vi "SimpleLiveAppHistogram.vi"() -> ()   [LabVIEW 2018]
uses:
  D:/SVN/PM/sdk/AppSamples/LabVIEWSamples/trunk/Release/2018/Dependencies/PVCamNET.dll
  Dependencies/PVCamNET.dll
  CommonFiles/GlobalVariables.vi
panel:
  out "Capturing":bool
  in  "Histogram On/Off":bool
  out "8 Bit Histogram":i32[](graph)
  in  "Exposure Time":dbl
  out "Live":bool
  out "Camera Status":bool
  in  "Uninit":bool
  in  "Live stop":bool
  in  "Live start":bool
  in  "Init":bool
  # "SimpleLiveAppHistogram.vi\n\nDescription:\nThis sample code lets the user use live mode in an event driven structure.\nDuring live mode the user is able to turn on and off 8 bit histogram.\n\nSteps to run:\n1. Click \"Run\"\n2. Click \"Open\"\n3. Enter Exposure Time\n4. Click \"Live start\"\n5. Click Histogram toggle switch\n6. Click \"Live stop\"\n7. Click \"Close\""
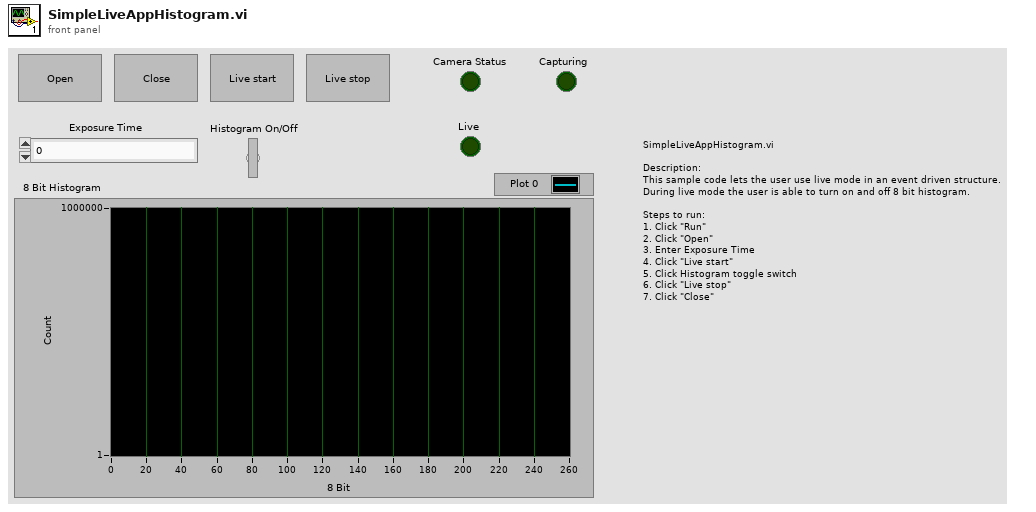
[diagram p1: front panel]
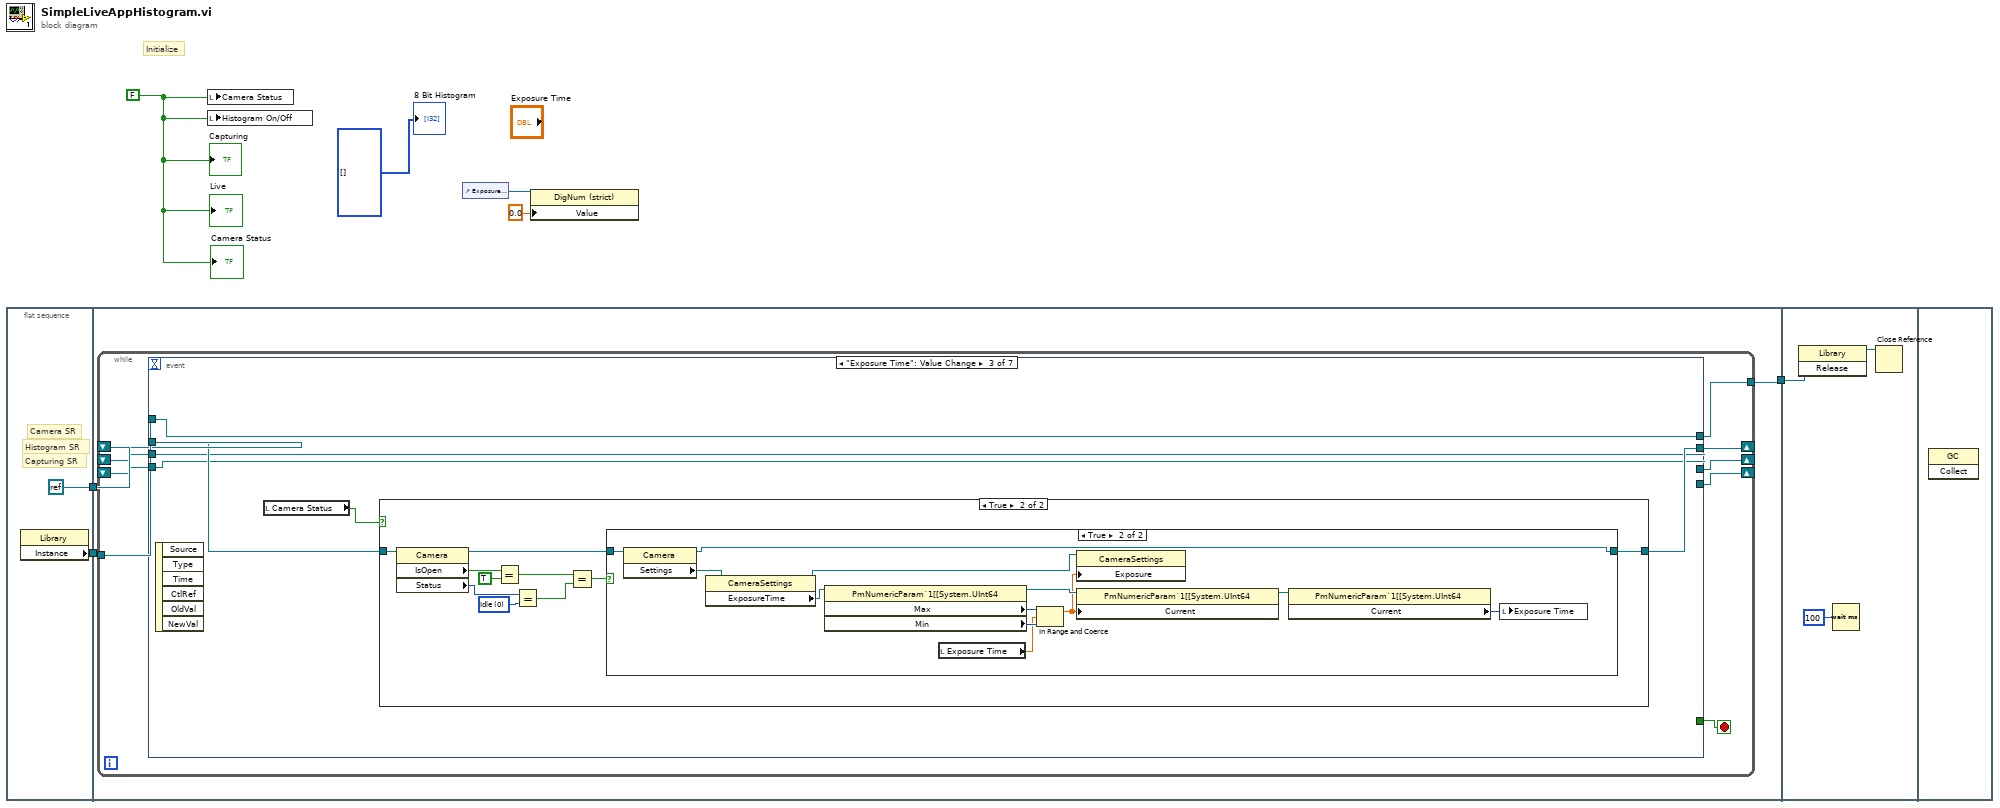
[diagram p0: block diagram]
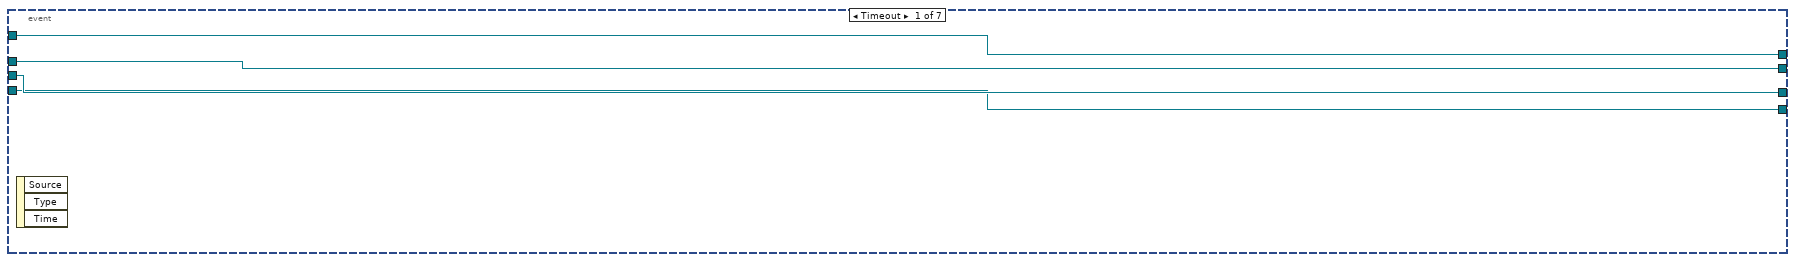
[diagram p2: hidden frame]
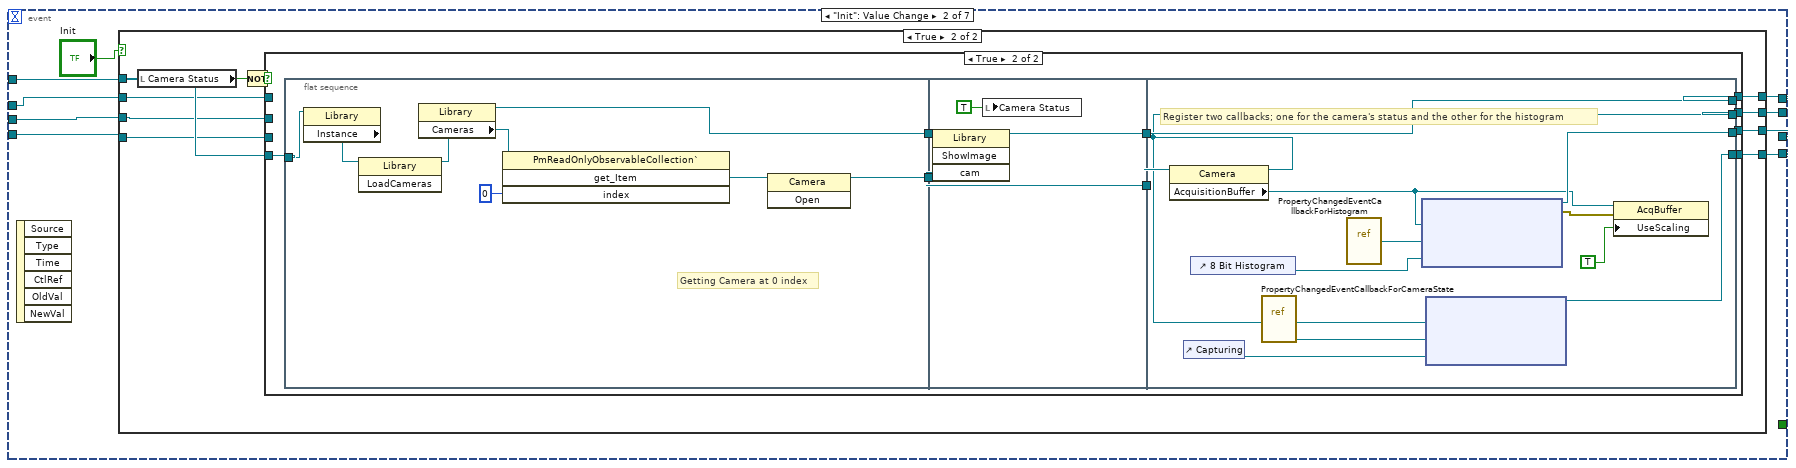
[diagram p3: hidden frame]
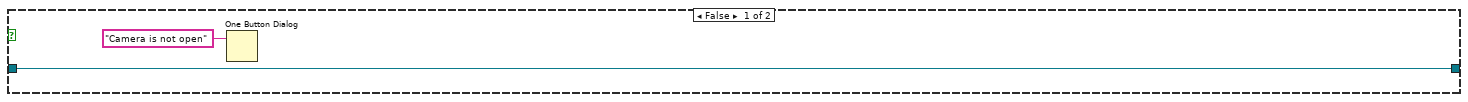
[diagram p6: hidden frame]
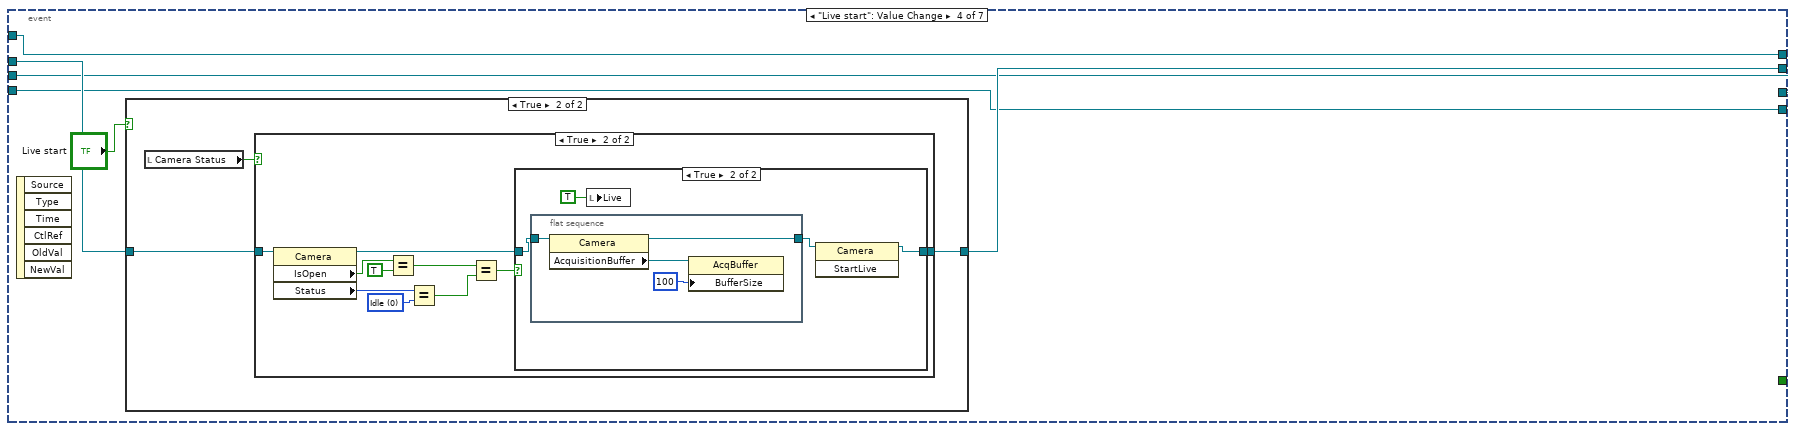
[diagram p8: hidden frame]
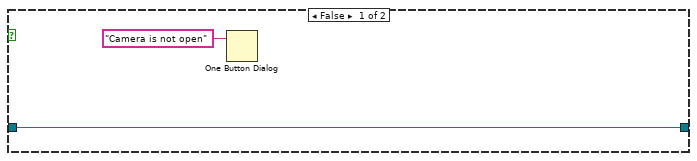
[diagram p10: hidden frame]
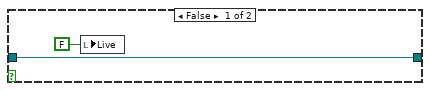
[diagram p11: hidden frame]
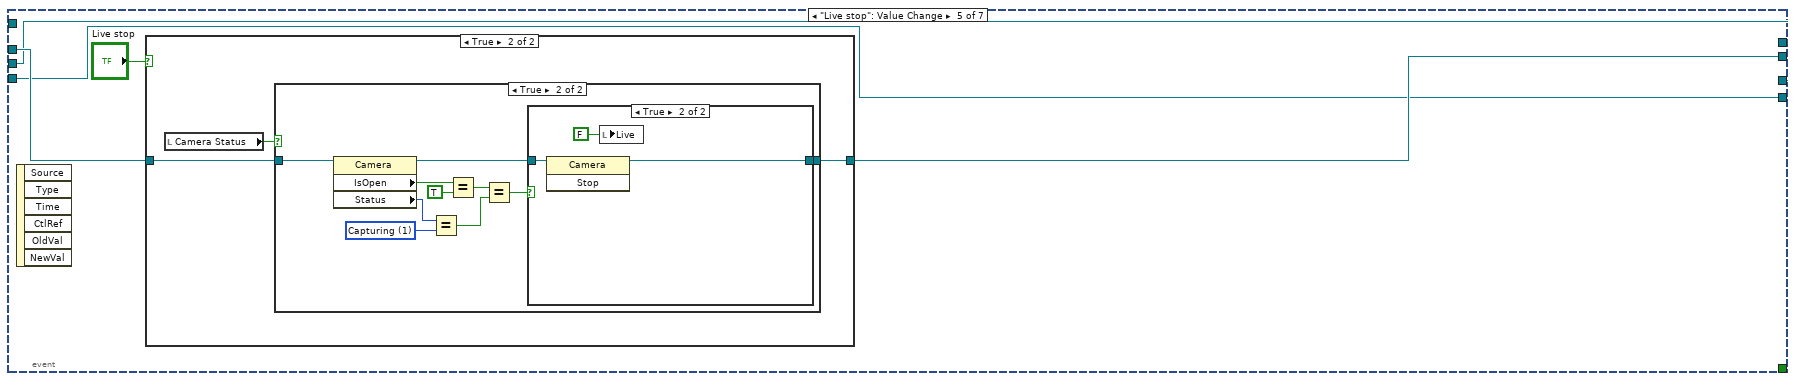
[diagram p12: hidden frame]
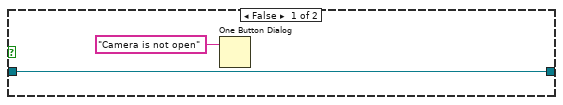
[diagram p14: hidden frame]
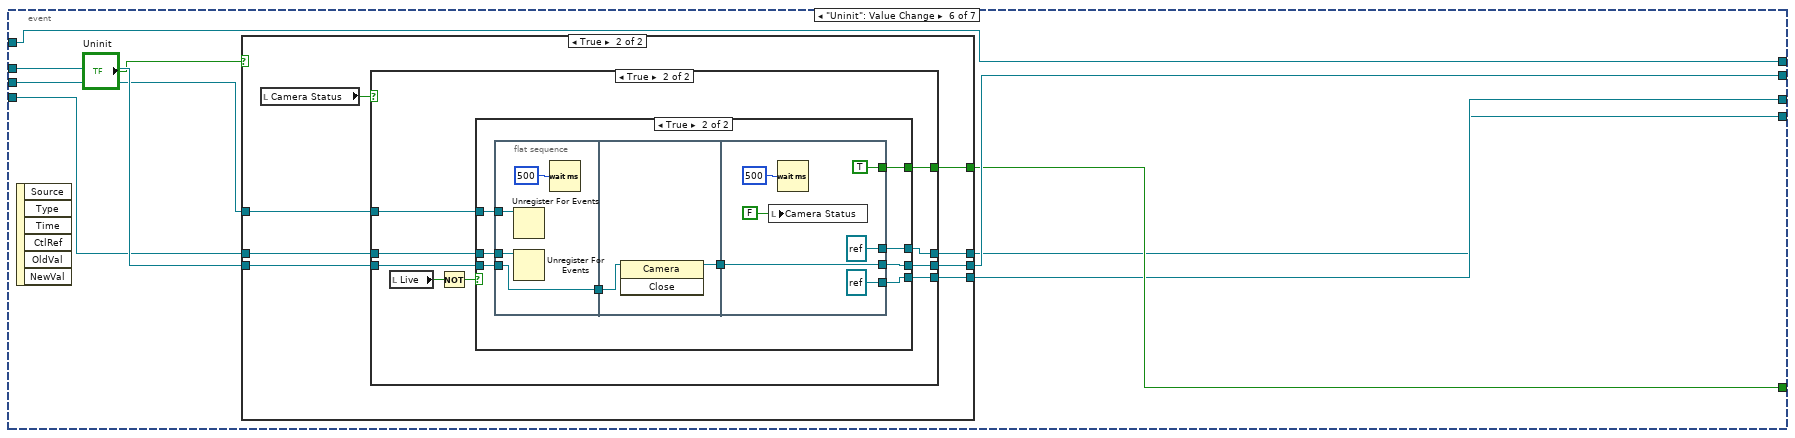
[diagram p16: hidden frame]
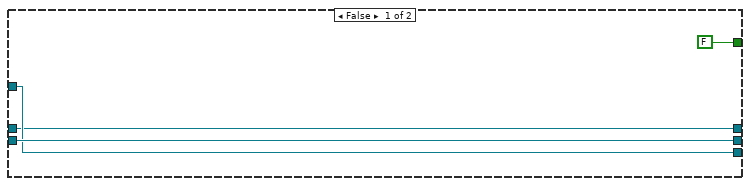
[diagram p17: hidden frame]
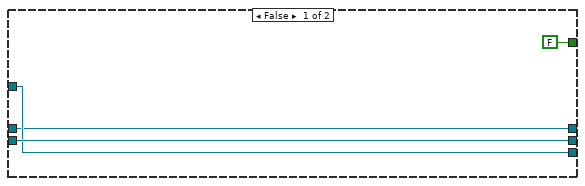
[diagram p18: hidden frame]
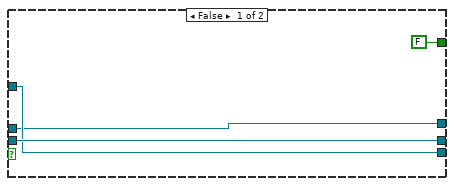
[diagram p19: hidden frame]
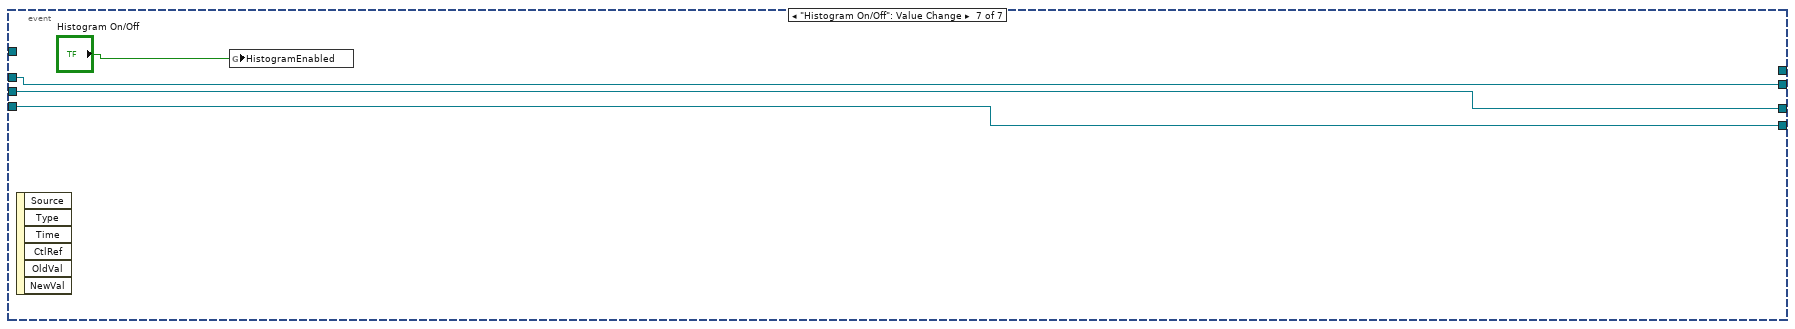
[diagram p20: hidden frame]
diagram:
  w3 = FALSE ("Histogram On/Off")
  # "Initialize"
  n1 = flat-sequence {
    tunnel: [w9] -> w7
    tunnel: [refnum<k0> refnum] -> w5
    tunnel: w7 -> [w12]
    tunnel: [w11] -> w6
    tunnel: w5 -> [w10]
    tunnel: w6 -> [w238]
    frame #0 {
      # "Histogram SR"
      # "Camera SR"
      # "Capturing SR"
      n2 = property class="Library"() -> ("Instance"=w9:refnum<k24>)  [unwired: 2 in, 2 out]
    }
    frame #1 {
      n3 = while {
        tunnel: w12 -> [w21]
        shift-right: [w20] -> _
        shift-left: w10 -> [w17]
        tunnel: [w19] -> w11
        shift-right: [w16] -> _
        shift-left: _ -> [w15]
        shift-right: [w14] -> _
        shift-left: _ -> [w13]
        stop <- w18 stop-if-true
        n4 = event shown="[2] \"Exposure Time\": Value Change" {
          selector: _ -> [_ _ _ _ _ _ _]
          dyn-events: _ -> [_ _ _ _ _ _ _]
          timeout: _ -> [_ _ _ _ _ _ _]
          tunnel: w21 -> [w24 w34 w89 w120 _ w180 _]
          tunnel: [w25 w33 w90 w119 w151 w181 w235] -> w20
          tunnel: [w24 w32 w89 w120 _ w180 _] -> w19
          tunnel: w17 -> [w25 w31 w91 w121 w152 w182 w235]
          tunnel: [_ _ _ _ _ w179 _] -> w18
          tunnel: [w23 w29 w87 w118 w150 w177 w236] -> w16
          tunnel: w15 -> [w23 w28 w87 w118 w150 w178 w236]
          tunnel: [w22 w27 w86 w117 w149 w174 w233] -> w14
          tunnel: w13 -> [w22 w26 w86 w117 w149 w175 w233]
          event Timeout {
            n5 = event-data() -> ()  [unwired: 1 in, 3 out]
          }
          event "Init": Value Change {
            n6 = event-data() -> ()  [unwired: 1 in, 6 out]
            n7 = case shown="True" "Init" {
              tunnel: w34 -> [w38 w48]
              tunnel: [w37 w47] -> w33
              tunnel: [w38 w46] -> w32
              tunnel: w31 -> [w37 w43]
              tunnel: [w36 w42] -> w29
              tunnel: w28 -> [w36 w41]
              tunnel: [w35 w40] -> w27
              tunnel: w26 -> [w35 w39]
              frame False {
              }
              frame True {
                n8 = local read "Camera Status"() -> (w45:bool)
                n9 = Not(x=w45) -> (.not. x?=w44:bool)
                n10 = case shown="True" w44 {
                  tunnel: w48 -> [w51 w59]
                  tunnel: [w52 w58] -> w47
                  tunnel: [w51 w57] -> w46
                  tunnel: w43 -> [w52 _]
                  tunnel: [w50 w54] -> w42
                  tunnel: w41 -> [w50 _]
                  tunnel: [w49 w53] -> w40
                  tunnel: w39 -> [w49 _]
                  frame False {
                  }
                  frame True {
                    n11 = flat-sequence {
                      tunnel: w59 -> [w64]
                      tunnel: [w66] -> w61
                      tunnel: [w65] -> w60
                      tunnel: w61 -> [w72]
                      tunnel: w60 -> [w73]
                      tunnel: [w73] -> w56
                      tunnel: [w71] -> w55
                      tunnel: [w85] -> w57
                      tunnel: [w79] -> w58
                      tunnel: w56 -> [w84]
                      tunnel: w55 -> [w85]
                      tunnel: [w83] -> w54
                      tunnel: [w78] -> w53
                      frame #0 {
                        # "Getting Camera at 0 index"
                        n12 = property class="Library"(reference=w64) -> ("Instance"=w63:refnum<k24>)  [unwired: 1 in, 2 out]
                        n13 = invoke class="Library" method="LoadCameras"(reference=w63) -> (reference out=w62:refnum<k24>)  [unwired: 2 in, 2 out]
                        n14 = property class="Library"(reference=w62) -> (reference out=w66:refnum<k24>, "Cameras"=w69:refnum<k24>)  [unwired: 1 in, 1 out]
                        n15 = invoke class="PmReadOnlyObservableCollection`" method="get_Item"(reference=w69, "index"=0) -> ("get_Item"=w67:refnum<k24>)  [unwired: 2 in, 3 out]
                        n16 = invoke class="Camera" method="Open"(reference=w67) -> (reference out=w65:refnum<k24>)  [unwired: 2 in, 2 out]
                      }
                      frame #1 {
                        n17 = invoke class="Library" method="ShowImage"(reference=w72, "cam"=w73) -> (reference out=w71:refnum<k24>)  [unwired: 2 in, 3 out]
                        n18 = local write "Camera Status"(TRUE ("Camera Status")) -> ()
                      }
                      frame #2 {
                        # "Register two callbacks; one for the camera's status and the other for the histogram"
                        n19 = property class="Camera"(reference=w84) -> (reference out=w79:refnum<k24>, "AcquisitionBuffer"=w75:refnum<k24>)  [unwired: 1 in, 1 out]
                        n20 = control-ref of="Capturing"() -> (w80:refnum<vi>)
                        n21 = control-ref of="8 Bit Histogram"() -> (w82:refnum<vi>)
                        n22 = vi-ref "PropertyChangedEventCallbackForCameraState.vi"() -> ("vi reference"=w77:refnum<vi>)
                        n23 = vi-ref "PropertyChangedEventCallbackForHistogram.vi"() -> ("vi reference"=w81:refnum<vi>)
                        n24 = node(w75, w81, w82) -> (w83:refnum<k27>, w76:errorcluster)  [unwired: 2 in]
                        n25 = node(w79, w77, w80) -> (w78:refnum<k27>)  [unwired: 2 in, 1 out]
                        n26 = property class="AcqBuffer"(reference=w75, error in=w76, "UseScaling"=TRUE) -> ()  [unwired: 2 out]
                      }
                    }
                  }
                }
              }
            }
          }
          event "Exposure Time": Value Change {
            n27 = event-data() -> ()  [unwired: 1 in, 6 out]
            n28 = local read "Camera Status"() -> (w88:bool)
            n29 = case shown="True" w88 {
              tunnel: w91 -> [w93 w97]
              tunnel: [w93 w94] -> w90
              frame False {
                n30 = One Button Dialog(message="Camera is not open") -> ()  [unwired: 1 in, 1 out]
              }
              frame True {
                w102 = 0 items=["Idle", "Capturing"] ("Status")
                n31 = property class="Camera"(reference=w97) -> (reference out=w95:refnum<k24>, "IsOpen"=w101:bool, "Status"=w103:i32)  [unwired: 1 in, 1 out]
                n32 = Equal?(x=w101, y=TRUE) -> (x = y?=w99:bool)
                n33 = Equal?(x=w103, y=w102) -> (x = y?=w98:bool)
                n34 = Equal?(x=w99, y=w98) -> (x = y?=w96:bool)
                n35 = case shown="True" w96 {
                  tunnel: w95 -> [w104 w116]
                  tunnel: [w104 w108] -> w94
                  frame False {
                  }
                  frame True {
                    n36 = property class="Camera"(reference=w116) -> (reference out=w108:refnum<k24>, "Settings"=w107:refnum<k24>)  [unwired: 1 in, 1 out]
                    n37 = property class="CameraSettings"(reference=w107) -> (reference out=w106:refnum<k24>, "ExposureTime"=w105:refnum<k24>)  [unwired: 1 in, 1 out]
                    n38 = property class="PmNumericParam`1[[System.UInt64"(reference=w105) -> (reference out=w113:refnum<k24>, "Max"=w115:u64, "Min"=w114:u64)  [unwired: 1 in, 1 out]
                    n39 = local read "Exposure Time"() -> (w110:dbl)
                    n40 = In Range and Coerce(upper limit=w115, x=w110, lower limit=w114) -> (coerced(x)=w111:dbl)  [unwired: 1 out]
                    n41 = property class="CameraSettings"(reference=w106, "Exposure"=w111) -> ()  [unwired: 1 in, 2 out]
                    n42 = property class="PmNumericParam`1[[System.UInt64"(reference=w113, "Current"=w111) -> (reference out=w112:refnum<k24>)  [unwired: 1 in, 1 out]
                    n43 = property class="PmNumericParam`1[[System.UInt64"(reference=w112) -> ("Current"=w109:u64)  [unwired: 1 in, 2 out]
                    n44 = local write "Exposure Time"(w109) -> ()
                  }
                }
              }
            }
          }
          event "Live start": Value Change {
            n45 = event-data() -> ()  [unwired: 1 in, 6 out]
            n46 = case shown="True" "Live start" {
              tunnel: w121 -> [w123 w126]
              tunnel: [w123 w125] -> w119
              frame False {
              }
              frame True {
                n47 = local read "Camera Status"() -> (w124:bool)
                n48 = case shown="True" w124 {
                  tunnel: w126 -> [w127 w132]
                  tunnel: [w127 w130] -> w125
                  frame False {
                    n49 = One Button Dialog(message="Camera is not open") -> ()  [unwired: 1 in, 1 out]
                  }
                  frame True {
                    w137 = 0 items=["Idle", "Capturing"] ("Status")
                    n50 = property class="Camera"(reference=w132) -> (reference out=w131:refnum<k24>, "IsOpen"=w136:bool, "Status"=w138:i32)  [unwired: 1 in, 1 out]
                    n51 = Equal?(x=w136, y=TRUE) -> (x = y?=w134:bool)
                    n52 = Equal?(x=w138, y=w137) -> (x = y?=w133:bool)
                    n53 = Equal?(x=w134, y=w133) -> (x = y?=w129:bool)
                    n54 = case shown="True" w129 {
                      tunnel: w131 -> [w140 w142]
                      tunnel: [w140 w143] -> w130
                      frame False {
                        n55 = local write "Live"(FALSE ("Live 2")) -> ()
                      }
                      frame True {
                        n56 = flat-sequence {
                          tunnel: w142 -> [w148]
                          tunnel: [w147] -> w141
                          frame #0 {
                            n57 = property class="Camera"(reference=w148) -> (reference out=w147:refnum<k24>, "AcquisitionBuffer"=w146:refnum<k24>)  [unwired: 1 in, 1 out]
                            n58 = property class="AcqBuffer"(reference=w146, "BufferSize"=100) -> ()  [unwired: 1 in, 2 out]
                          }
                        }
                        n59 = local write "Live"(TRUE ("Live")) -> ()
                        n60 = invoke class="Camera" method="StartLive"(reference=w141) -> (reference out=w143:refnum<k24>)  [unwired: 2 in, 2 out]
                      }
                    }
                  }
                }
              }
            }
          }
          event "Live stop": Value Change {
            n61 = event-data() -> ()  [unwired: 1 in, 6 out]
            n62 = case shown="True" "Live stop" {
              tunnel: w152 -> [w154 w157]
              tunnel: [w154 w156] -> w151
              frame False {
              }
              frame True {
                n63 = local read "Camera Status"() -> (w155:bool)
                n64 = case shown="True" w155 {
                  tunnel: w157 -> [w159 w169]
                  tunnel: [w159 w166] -> w156
                  frame False {
                    n65 = One Button Dialog(message="Camera is not open") -> ()  [unwired: 1 in, 1 out]
                  }
                  frame True {
                    w164 = 1 items=["Idle", "Capturing"] ("Status")
                    n66 = property class="Camera"(reference=w169) -> (reference out=w167:refnum<k24>, "IsOpen"=w163:bool, "Status"=w165:i32)  [unwired: 1 in, 1 out]
                    n67 = Equal?(x=w165, y=w164) -> (x = y?=w160:bool)
                    n68 = Equal?(x=w163, y=TRUE) -> (x = y?=w161:bool)
                    n69 = Equal?(x=w161, y=w160) -> (x = y?=w168:bool)
                    n70 = case shown="True" w168 {
                      tunnel: w167 -> [w170 w173]
                      tunnel: [w170 w172] -> w166
                      frame False {
                      }
                      frame True {
                        n71 = invoke class="Camera" method="Stop"(reference=w173) -> (reference out=w172:refnum<k24>)  [unwired: 2 in, 2 out]
                        n72 = local write "Live"(FALSE ("Live 2")) -> ()
                      }
                    }
                  }
                }
              }
            }
          }
          event "Uninit": Value Change {
            n73 = event-data() -> ()  [unwired: 1 in, 6 out]
            n74 = case shown="True" "Uninit" {
              tunnel: w182 -> [w186 w194]
              tunnel: [w186 w193] -> w181
              tunnel: [FALSE ("Camera Status") w191] -> w179
              tunnel: w178 -> [w184 w190]
              tunnel: [w184 w189] -> w177
              tunnel: w175 -> [w183 w188]
              tunnel: [w183 w187] -> w174
              frame False {
              }
              frame True {
                n75 = local read "Camera Status"() -> (w192:bool)
                n76 = case shown="True" w192 {
                  tunnel: w194 -> [w198 w207]
                  tunnel: [w198 w206] -> w193
                  tunnel: [FALSE ("Camera Status") w205] -> w191
                  tunnel: w190 -> [w196 w202]
                  tunnel: [w196 w201] -> w189
                  tunnel: w188 -> [w195 w200]
                  tunnel: [w195 w199] -> w187
                  frame False {
                  }
                  frame True {
                    n77 = local read "Live"() -> (w203:bool)
                    n78 = Not(x=w203) -> (.not. x?=w204:bool)
                    n79 = case shown="True" w204 {
                      tunnel: w207 -> [w211 w219]
                      tunnel: [w211 w218] -> w206
                      tunnel: [FALSE ("Camera Status") w217] -> w205
                      tunnel: w202 -> [w209 w215]
                      tunnel: [w209 w214] -> w201
                      tunnel: w200 -> [w208 w213]
                      tunnel: [w208 w212] -> w199
                      frame False {
                      }
                      frame True {
                        n80 = flat-sequence {
                          tunnel: w219 -> [w224]
                          tunnel: [w224] -> w216
                          tunnel: w215 -> [w223]
                          tunnel: w213 -> [w221]
                          tunnel: [w225] -> w220
                          tunnel: w216 -> [w226]
                          tunnel: [w232] -> w218
                          tunnel: w220 -> [w232]
                          tunnel: [TRUE ("Camera Status")] -> w217
                          tunnel: [refnum<k27> refnum ("Event Callback")] -> w214
                          tunnel: [refnum<k27> refnum ("Event Callback")] -> w212
                          frame #0 {
                            n81 = Unregister For Events(event registration refnum=w223) -> ()  [unwired: 1 in, 1 out]
                            n82 = Unregister For Events(event registration refnum=w221) -> ()  [unwired: 1 in, 1 out]
                            n83 = Wait (ms)(milliseconds to wait=u32 500) -> ()  [unwired: 1 out]
                          }
                          frame #1 {
                            n84 = invoke class="Camera" method="Close"(reference=w226) -> (reference out=w225:refnum<k24>)  [unwired: 2 in, 2 out]
                          }
                          frame #2 {
                            n85 = local write "Camera Status"(FALSE ("Camera Status")) -> ()
                            n86 = Wait (ms)(milliseconds to wait=u32 500) -> ()  [unwired: 1 out]
                          }
                        }
                      }
                    }
                  }
                }
              }
            }
          }
          event "Histogram On/Off": Value Change {
            n87 = event-data() -> ()  [unwired: 1 in, 6 out]
            n88 = global write "GlobalVariables.vi" "HistogramEnabled"("Histogram On/Off") -> ()
          }
        }
      }
    }
    frame #2 {
      n89 = invoke class="Library" method="Release"(reference=w238) -> (reference out=w239:refnum<k24>)  [unwired: 2 in, 2 out]
      n90 = Wait (ms)(milliseconds to wait=u32 100) -> ()  [unwired: 1 out]
      n91 = Close Reference(reference=w239) -> ()  [unwired: 1 in, 1 out]
    }
    frame #3 {
      n92 = invoke class="GC" method="Collect"() -> ()  [unwired: 3 in, 3 out]
    }
  }
  n93 = local write "Camera Status"(w3) -> ()
  n94 = local write "Histogram On/Off"(w3) -> ()
  n95 = control-ref of="Exposure Time"() -> (w2:refnum<vi>)
  n96 = property class="DigNum (strict)"(reference=w2, "Value"=0.0) -> ()  [unwired: 1 in, 2 out]
  "Camera Status" <- w3
  "Live" <- w3
  "8 Bit Histogram" <- i32[] [] ("8 Bit Histogram")
  "Capturing" <- w3
